vi "拉取dll.vi"(9 "MD5 message-digest":string="47126f942acc1a6f17c5325a05c10f2e", 10 "名称或相对路径":string="FreeMem.dll", 11 "服务器":T1={"host"="27.154.58.30", "port"=8020, "user"="std", "password"="std23506", "远端地址"="/微站/四代/一体化微型水质监测站.exe"}) -> (0 "error out":errorcluster caption="错误输出")   [LabVIEW 2016, in "update.lvlib"]
uses:
  update.lvlib
  <vilib>/httpClient/POSTBuffer.vi
  <vilib>/httpClient/LabVIEWHTTPClient.lvlib
panel:
  out "headers":string caption="头部"
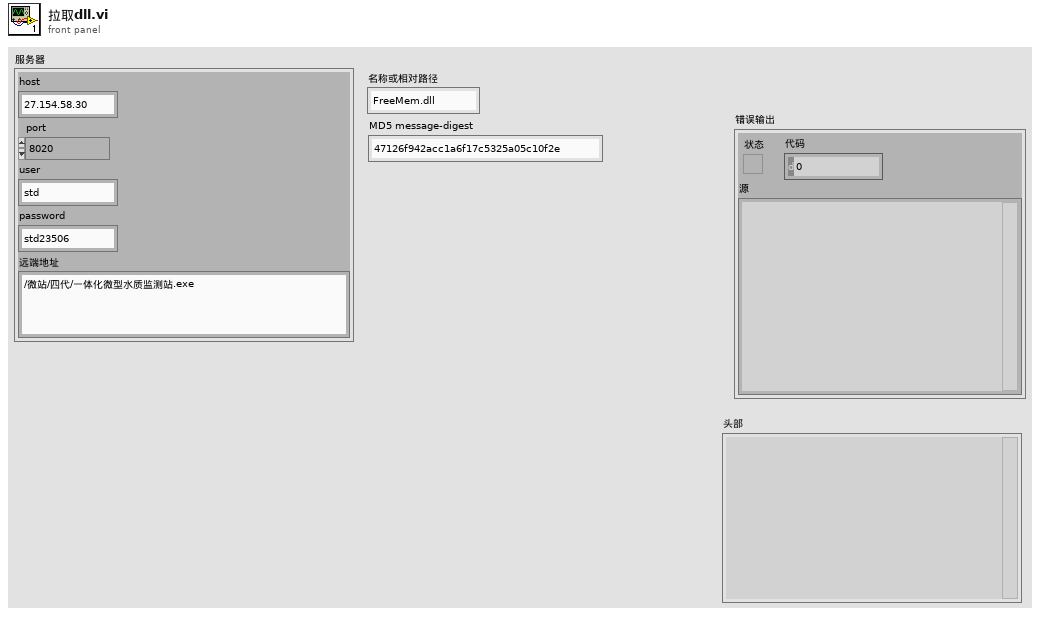
[diagram p1: front panel]
types:
  T1 = cluster{"host":string, "port":u16, "user":string, "password":string, "远端地址":string}
  T2 = typedef "LabVIEWHTTPClient.lvlib/ClientHandle.ctl" = refnum<k1>
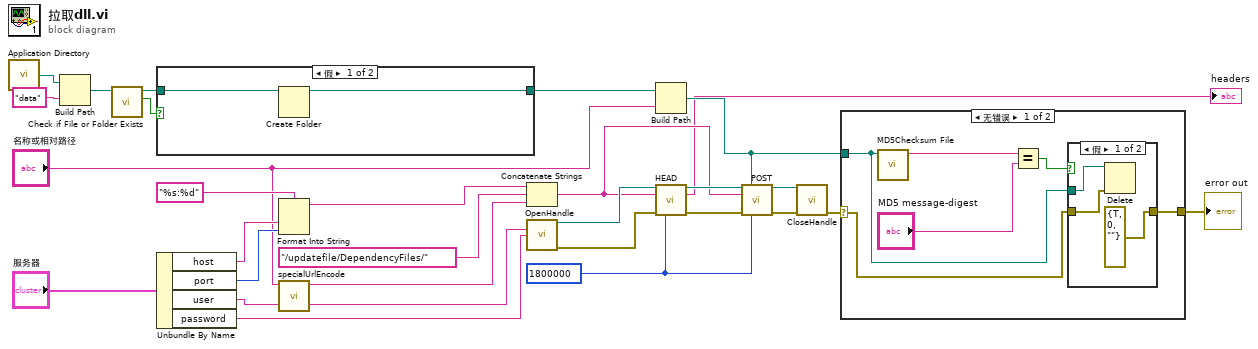
[diagram p0: block diagram]
diagram:
  w15 = 1800000 ("timeout (10000)")
  n1 = call <vilib>:"Application Directory.vi"() -> ("Application Directory"=w8:path)
  n2 = Build Path(base path=w8, name or relative path="data" ("名称或相对路径")) -> (appended path=w9:path)
  n3 = call <vilib>:"Check if File or Folder Exists.vi"("path"=w9) -> ("file or folder exists?"=w10:bool, "dup path"=w11:path)  [unwired: 8 in, 1 out]
  n4 = case shown="假" w10 {
    tunnel: w11 -> [w30 w31]
    tunnel: [w29 w31] -> w6
    frame False {
      n5 = Create Folder(path (use dialog)=w30) -> (created path=w29:path)  [unwired: 2 in, 2 out]
    }
    frame True {
    }
  }
  n6 = Unbundle By Name("服务器") -> ("host"=w26:string, "port"=w25:u16, "user"=w14:string, "password"=w13:string)
  n7 = Format Into String(format string="%s:%d" ("格式字符串"), w26, w25) -> (resulting string=w23:string)  [unwired: 2 in, 1 out]
  n8 = call "specialUrlEncode.vi"("str"="名称或相对路径") -> ("UrlEncode"=w22:string)  [unwired: 10 in]
  n9 = Concatenate Strings(w23, "/updatefile/DependencyFiles/", w22) -> (w12:string)
  n10 = call <vilib>:"OpenHandle.vi"("username"=w14, "password"=w13) -> ("client handle out"=w19:T2, "error out"=w17:errorcluster)  [unwired: 12 in]
  n11 = Build Path(base path=w6, name or relative path="名称或相对路径") -> (appended path=w4:path)
  n12 = call <vilib>:"HEAD.vi"("client handle"=w19, "url"=w12, "error in (no error)"=w17, "timeout (10000)"=w15) -> ("client handle out"=w18:T2, "headers"=→"headers":string, "error out"=w16:errorcluster)  [unwired: 9 in]
  n13 = call-poly <vilib>:"POST.vi"("client handle"=w18, "output file"=w4, "url"=w12, "error in (no error)"=w16, "timeout (10000)"=w15) -> ("client handle out"=w21:T2, "error out"=w20:errorcluster)  [unwired: 7 in, 2 out]
  n14 = call <vilib>:"CloseHandle.vi"("client handle"=w21, "error in (no error)"=w20) -> ("error out"=w5:errorcluster)  [unwired: 13 in]
  n15 = case shown="无错误" w5 {
    selector: w5 -> [w35 w42]
    tunnel: w4 -> [w33 _]
    tunnel: [w34 w42] -> w3
    frame No Error {
      n16 = call <vilib>:"MD5Checksum File.vi"("Path"=w33) -> ("MD5 message-digest"=w37:string)  [unwired: 9 in, 1 out]
      n17 = Equal?(x=w37, y="MD5 message-digest") -> (x = y?=w36:bool)
      n18 = case shown="假" w36 {
        tunnel: w35 -> [w38 w41]
        tunnel: [errorcluster {"status"=TRUE, "code"=0, "source"=""} ("error IO") w41] -> w34
        tunnel: w33 -> [w39 _]
        frame False {
          n19 = Delete(path (use dialog)=w39, error in=w38) -> ()  [unwired: 3 in, 3 out]
        }
        frame True {
        }
      }
    }
    frame Error {
    }
  }
  "error out" <- w3
